vi "Build.vi"(5 "HttpRequestMessage in":refnum<class "HttpRequestMessage.lvclass">, 8 "error in (no error)":errorcluster, 11 "HttpRequestMessage":refnum<k24>) -> (0 "error out":errorcluster, 3 "HttpRequestMessage out":refnum<class "HttpRequestMessage.lvclass">)   [LabVIEW 2018, in "HttpClient_NET.lvlib" / "HttpRequestMessage.lvclass"]
doc: "<b> </b> <b> </b>\nHttpClient_NET\nJustin Young - Viviota\nCopyright (c) 2021\nLicense: BSD"
uses:
  HttpRequestMessage.lvclass
  System.Net.Http
  HttpRequestMessage.lvclass/HttpRequestMessage.ctl
  Accessors/Write NET_HttpRequestMessage.vi
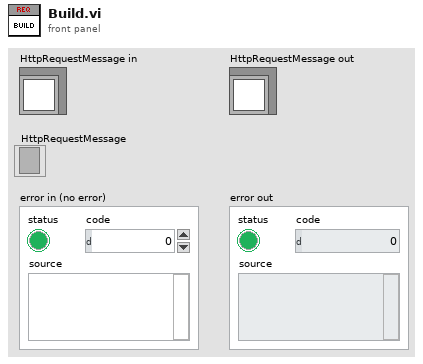
[diagram p1: front panel]
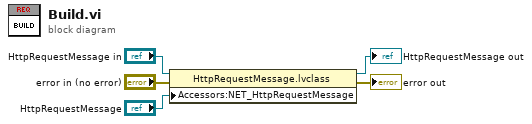
[diagram p0: block diagram]
diagram:
  n1 = property class="HttpRequestMessage.lvclass"(reference="HttpRequestMessage in", error in="error in (no error)", "Accessors:NET_HttpRequestMessage"="HttpRequestMessage") -> (reference out=→"HttpRequestMessage out":refnum<class "HttpRequestMessage.lvclass">, error out=→"error out":errorcluster)
